vi "Keithley 2600 Series Current Sweep Script.vi"() -> ()   [LabVIEW 2019, in "Keithley 2600 Series.lvlib"]
doc: "This example shows how to create, run a script and query the script output data."
uses:
  Keithley 2600 Series.lvlib
panel:
  out "Last Measured Voltage (V)":dbl
  out "Voltage Measurements (V)":string
  in  "Source Code":string="smua.reset()\nsmua.source.limitv = 1\nSweepILinMeasureV(smua, 0.01, 0.1, 0.2, 10)\nprintbuffer(1, 10, smua.nvbuffer1)\nprint(smua.nvbuffer1.readings[10])\n"
  in  "Script Variable (myScript)":string="myScript"
  in  "VISA resource name":refnum<visa-resource-name>
  # "(c) 2020 - 2022 National Instruments.  ALL RIGHTS RESERVED."
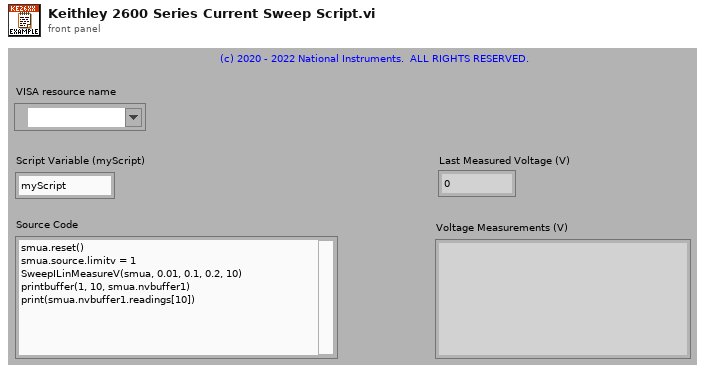
[diagram p1: front panel]
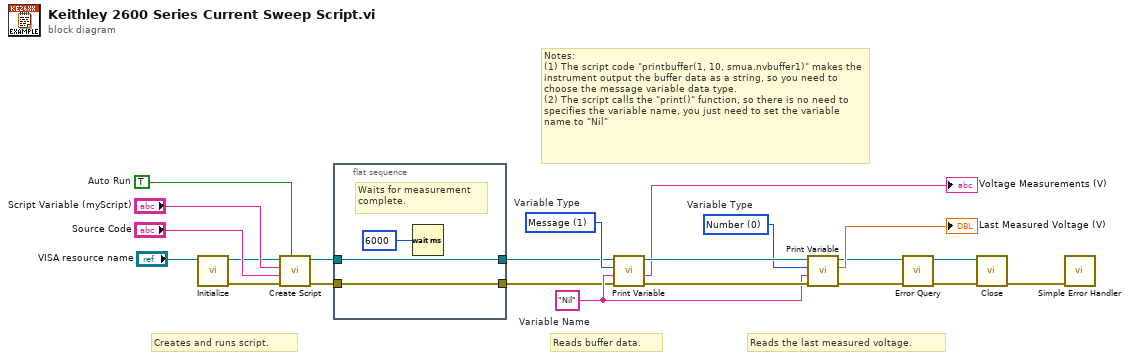
[diagram p0: block diagram]
diagram:
  w15 = 0 items=["Number", "Message"]  # Variable Type
  w18 = 1 items=["Number", "Message"]  # Variable Type
  w14 = "Nil"  # Variable Name
  w19 = TRUE  # Auto Run
  # "Reads buffer data."
  # "Reads the last measured voltage."
  # "Notes: \n(1) The script code \"printbuffer(1, 10, smua.nvbuffer1)\" makes the instrument output the buffer data as a string, so you need to choose the message variable data type.\n(2) The script calls the \"print()\" function, so there is no need to specifies the variable name, you just need to set the variable name to \"Nil\""
  # "Creates and runs script."
  n1 = call "Initialize.vi"("VISA resource name"="VISA resource name") -> ("error out"=w1:errorcluster, "VISA resource name out"=w2:refnum<visa-resource-name>)  [unwired: 9 in]
  n2 = call "Create Script.vi"("Auto Run (F: Disable)"=w19, "error in (no error)"=w1, "Source Code"="Source Code", "Script Variable"="Script Variable (myScript)", "VISA resource name"=w2) -> ("error out"=w12:errorcluster, "VISA resource name out"=w13:refnum<visa-resource-name>)  [unwired: 5 in]
  n3 = flat-sequence {
    tunnel: w13 -> [w23]
    tunnel: w12 -> [w24]
    tunnel: [w24] -> w10
    tunnel: [w23] -> w11
    frame #0 {
      # "Waits for measurement complete."
      n4 = Wait (ms)(milliseconds to wait=6000) -> ()  [unwired: 1 out]
    }
  }
  n5 = call "Print Variable.vi"("error in (no error)"=w10, "Variable Name"=w14, "Variable Type (0: Number)"=w18, "VISA resource name"=w11) -> ("error out"=w16:errorcluster, "Message"=→"Voltage Measurements (V)":string, "VISA resource name out"=w17:refnum<visa-resource-name>)  [unwired: 4 in, 1 out]
  n6 = call "Print Variable.vi"("error in (no error)"=w16, "Variable Name"=w14, "Variable Type (0: Number)"=w15, "VISA resource name"=w17) -> ("error out"=w6:errorcluster, "Number"=→"Last Measured Voltage (V)":dbl, "VISA resource name out"=w7:refnum<visa-resource-name>)  [unwired: 4 in, 1 out]
  n7 = call "Error Query.vi"("error in (no error)"=w6, "VISA resource name"=w7) -> ("error out"=w4:errorcluster, "VISA resource name out"=w5:refnum<visa-resource-name>)  [unwired: 6 in, 2 out]
  n8 = call "Close.vi"("error in (no error)"=w4, "VISA resource name"=w5) -> ("error out"=w20:errorcluster)  [unwired: 9 in]
  n9 = call <vilib>:"Simple Error Handler.vi"("error in (no error)"=w20) -> ()  [unwired: 4 in, 5 out]
